vi "process.vi"(8 "error in (no error)":errorcluster, 11 "Server in":refnum<class "Server.lvclass">) -> (0 "error out":errorcluster, 3 "Server out":refnum<class "Server.lvclass">)   [LabVIEW 2013, in "MQTT Server.lvlib" / "Server.lvclass"]
uses:
  Server.lvclass
  Control Packets/ControlPacket/ControlPacket.lvclass
  Server.lvclass/Server.ctl
  Response -- cluster.ctl
panel:
  out "History":cluster{"class name":string, "time":timestamp}[](array[cluster])
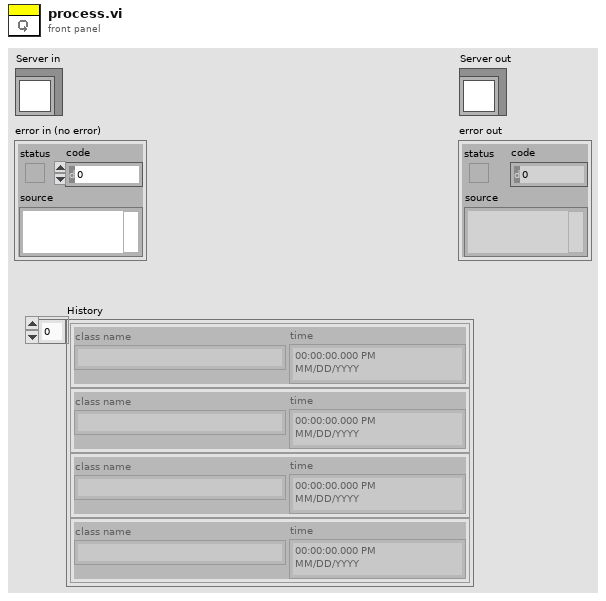
[diagram p1: front panel]
types:
  T1 = typedef "MQTT Server.lvlib/Server.lvclass/Response -- cluster.ctl" = cluster{"ServerResponse":refnum<class "ControlPacket.lvclass">, "Protocol Error":errorcluster}
  T2 = typedef "MQTT Server.lvlib/Server.lvclass/Request -- cluster.ctl" = cluster{"ServerRequest":refnum<class "ControlPacket.lvclass">, "SessionMailbox":refnum<queue>}
  T3 = cluster{"class name":string, "seconds since 1Jan1904":timestamp}
  T4 = cluster{"class name":string, "seconds since 1Jan1904":timestamp}[]
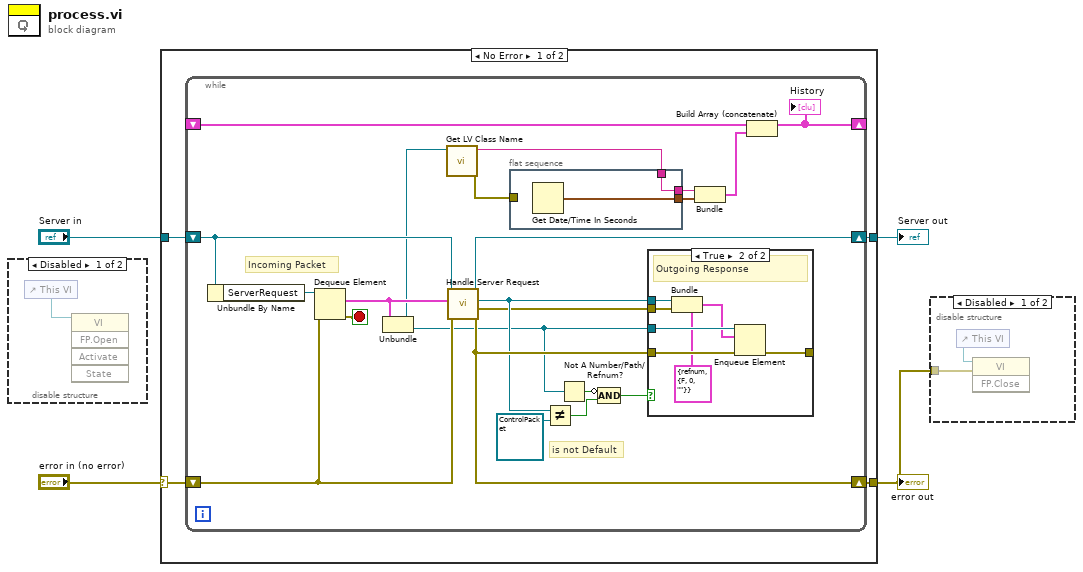
[diagram p0: block diagram]
diagram:
  n1 = disable-structure shown="Disabled" {
    frame Disabled {
      n2 = control-ref of="This VI"() -> (w5:refnum<vi>)
      n3 = invoke class="VI" method="FP.Open"(reference=w5) -> ()  [unwired: 4 in, 5 out]
    }
    frame Enabled {
    }
  }
  n4 = case shown="No Error" "error in (no error)" {
    selector: "error in (no error)" -> [w7 w42]
    tunnel: [w6 w42] -> w2
    tunnel: [w9 w41] -> w3
    tunnel: "Server in" -> [w8 w41]
    frame No Error {
      n5 = while {
        shift-right: [w30] -> w9
        shift-left: w8 -> [w29]
        shift-right: [w28] -> w6
        shift-left: w7 -> [w26]
        shift-right: [w19] -> _
        shift-left: _ -> [w21]
        stop <- w27 stop-if-true
        # "Incoming Packet"
        # "is not Default"
        n6 = Unbundle By Name(w29) -> ("ServerRequest"=w31:refnum<queue>)
        n7 = Dequeue Element(queue=w31, error in (no error)=w26) -> (element=w11:T2, error out=w27:errorcluster)  [unwired: 1 in, 2 out]
        n8 = Unbundle(w11) -> ("ServerRequest"=w10:refnum<class "ControlPacket.lvclass">, "SessionMailbox"=w16:refnum<queue>)
        n9 = call <vilib>:"Get LV Class Name.vi"("object"=w10) -> ("error out"=w25:errorcluster, "class name"=w24:string)  [unwired: 9 in]
        n10 = call-dynamic "Handle Server Request.vi"("error in (no error)"=w26, "Request"=w11, "Server in"=w29) -> ("error out"=w28:errorcluster, "Protocol Error"=w12:errorcluster, "ServerResponse"=w17:refnum<class "ControlPacket.lvclass">, "Server out"=w30:refnum<class "Server.lvclass">)  [unwired: 5 in]
        n11 = flat-sequence {
          tunnel: w25 -> [_]
          tunnel: w24 -> [w33]
          tunnel: [w33] -> w23
          tunnel: [w32] -> w22
          frame #0 {
            n12 = Get Date/Time In Seconds() -> (seconds since 1Jan1904=w32:timestamp)
          }
        }
        n13 = Not Equal?(x=w17, y=refnum<class "ControlPacket.lvclass"> refnum ("ControlPacket.lvclass")) -> (x != y?=w14:bool)
        n14 = Not A Number/Path/Refnum?(number/path/refnum=w16) -> (NaN/Path/Refnum?=w15:bool)
        n15 = Compound Arithmetic op=AND(invert w15, w14) -> (w13:bool)
        n16 = case shown="True" w13 {
          tunnel: w17 -> [_ w36]
          tunnel: w16 -> [_ w40]
          tunnel: w28 -> [_ w39]
          tunnel: [_ w38] -> _
          tunnel: w12 -> [_ w37]
          frame False {
          }
          frame True {
            # "Outgoing Response"
            n17 = Bundle(cluster=T1 {"ServerResponse"=refnum, "Protocol Error"={"status"=FALSE, "code"=0, "source"=""}} ("Response"), "ServerResponse"=w36, "Protocol Error"=w37) -> (w35:T1)
            n18 = Enqueue Element(queue=w40, element=w35, error in (no error)=w39) -> (error out=w38:errorcluster)  [unwired: 1 in, 2 out]
          }
        }
        n19 = Bundle("class name"=w23, "seconds since 1Jan1904"=w22) -> (w20:T3)  [unwired: 1 in]
        n20 = Build Array (concatenate)(w21, w20) -> (w19:T4)
        "History" <- w19
      }
    }
    frame Error {
    }
  }
  "error out" <- w2
  "Server out" <- w3
  n21 = disable-structure shown="Disabled" {
    disable-tunnel: w2 -> [w44 _]
    frame Disabled {
      n22 = control-ref of="This VI"() -> (w43:refnum<vi>)
      n23 = invoke class="VI" method="FP.Close"(reference=w43, error in=w44) -> ()  [unwired: 1 in, 3 out]
    }
    frame Enabled {
    }
  }
